vi "bits to string.vi"(10 "shift index":i32=4, 11 "bit stream":i8[](array[numeric])) -> (3 "string":string)   [LabVIEW 2013]
panel:
  out "Array":u8[](array[numeric])
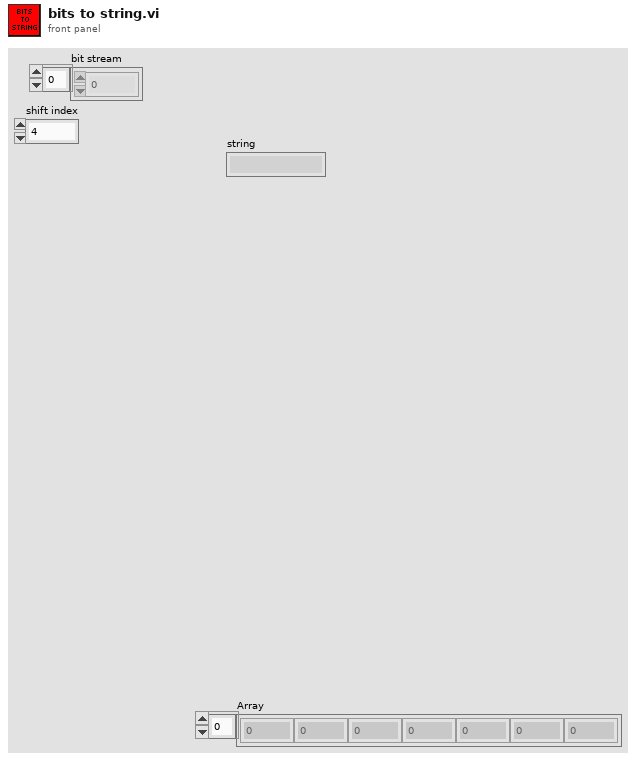
[diagram p1: front panel]
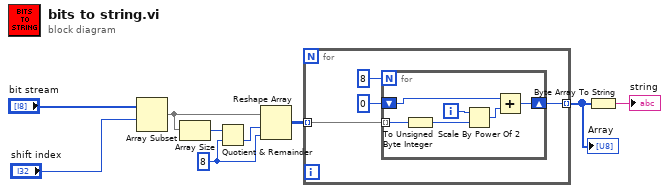
[diagram p0: block diagram]
diagram:
  w2 = 8 ("dimension size")
  n1 = Array Subset(array="bit stream", index="shift index") -> (w9:i8[])  [unwired: 1 in]
  n2 = Array Size(array=w9) -> (size(s)=w1:i32)
  n3 = Quotient & Remainder(x=w1, y=w2) -> (floor(x/y)=w3:i32)  [unwired: 1 out]
  n4 = Reshape Array(w9, w3, w2) -> (w4:i8[][])
  n5 = for {
    tunnel: w4 -> [w12] mode=indexing
    tunnel: [w11] -> w5 mode=indexing
    n6 = for {
      N: 8 -> [_]
      tunnel: w12 -> [w17] mode=indexing
      shift-right: [w18] -> w11
      shift-left: u8 0 -> [w14]
      i -> [w16]
      n7 = To Unsigned Byte Integer(number=w17) -> (unsigned 8bit integer=w15:u8)
      n8 = Scale By Power Of 2(n=w16, x=w15) -> (x*2^n=w19:u8)
      n9 = Add(x=w14, y=w19) -> (x+y=w18:u8)
    }
  }
  "Array" <- w5
  n10 = Byte Array To String(unsigned byte array=w5) -> (string=→"string":string)
